vi "Cal Amplitude and Phase.vi"(1 "Inst Types":T1[](array[typedef]), 6 "Channel ID":string[](array[string]), 7 "Test Ch Indices":i32[](array[numeric]), 8 "Reference Ch Index":i32) -> (0 "Valid Indices":i32[](array[numeric]), 3 "Ch Values":dbl[](array[numeric]), 5 "Ch Names":string[](array[string]))   [LabVIEW 2022 SP3]
uses:
  Controls/Inst_type.ctl
  Globals/Meas_global.vi
  <vilib>/measure/matone.llb/Extract Single Tone Information 1 Chan.vi
  <vilib>/measure/NI_MAPro.lvlib
panel:
  out "Ref Freq FFT":dbl
  out "detected frequency Ref":dbl format="%.2p"
  out "detected frequency":dbl format="%.2p"
  out "Ref Freq Hz Tone":dbl
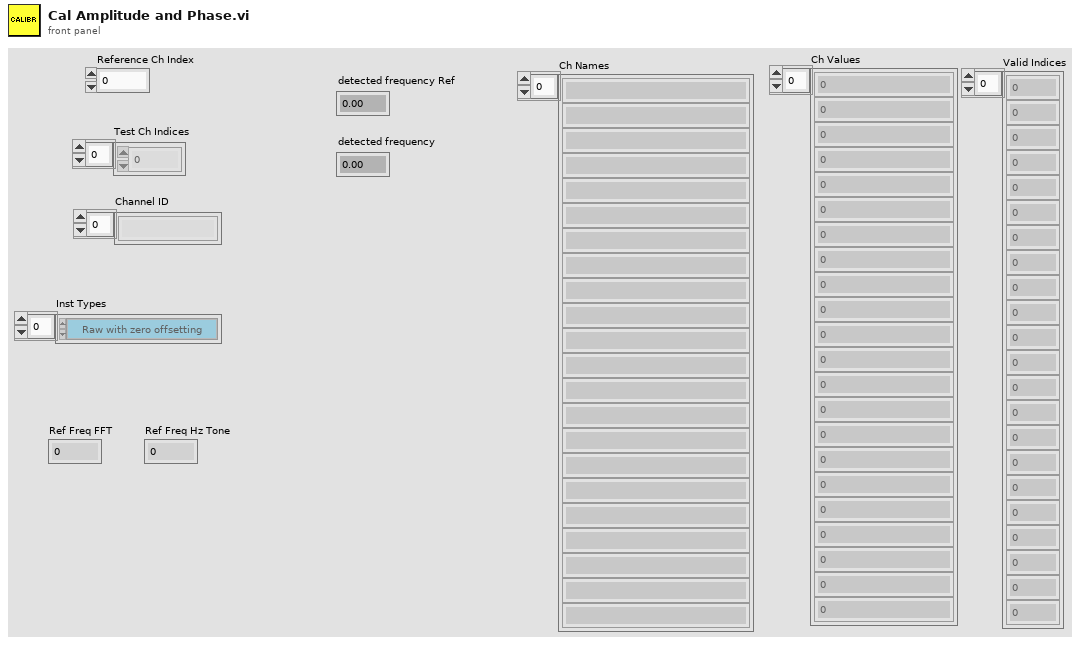
[diagram p1: front panel]
types:
  T1 = typedef "Inst_type.ctl" = enum16{"Raw voltage", "Raw with zero offsetting", "Propeller anemometer", "Pressure Transducer", "Pitot-static tube", "Hot wire", "Cross wire 1", "Cross wire 2", "Generic Linear", "Generic Polynomial", "Generic BackPoly", "Fast FID", "Thermocouple", "Cold wire", "Pulsed Wire", "LDA Vel", "LDA Tran time", "LDA Arr time", "Microphone"}
  T2 = typedef "Time_Trace_Cluster.ctl" = cluster{"Weighting":dbl[], "Voltage":dbl[], "Eng Values":dbl[]}
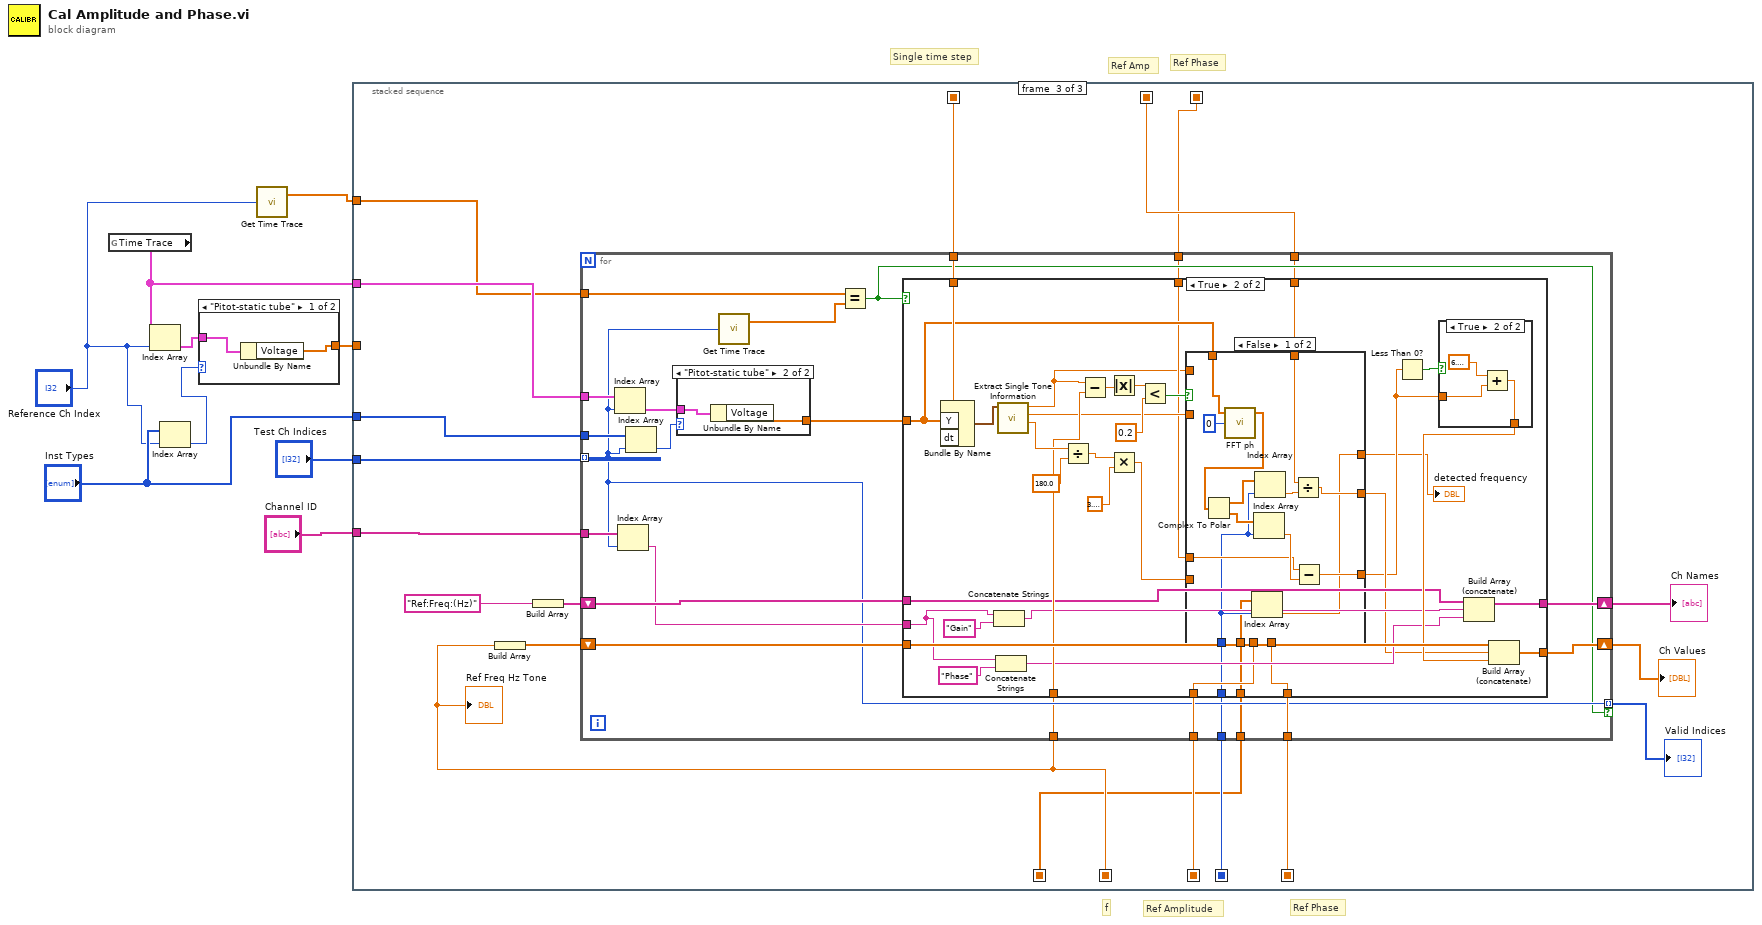
[diagram p0: block diagram]
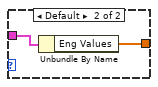
[diagram p2: hidden frame]
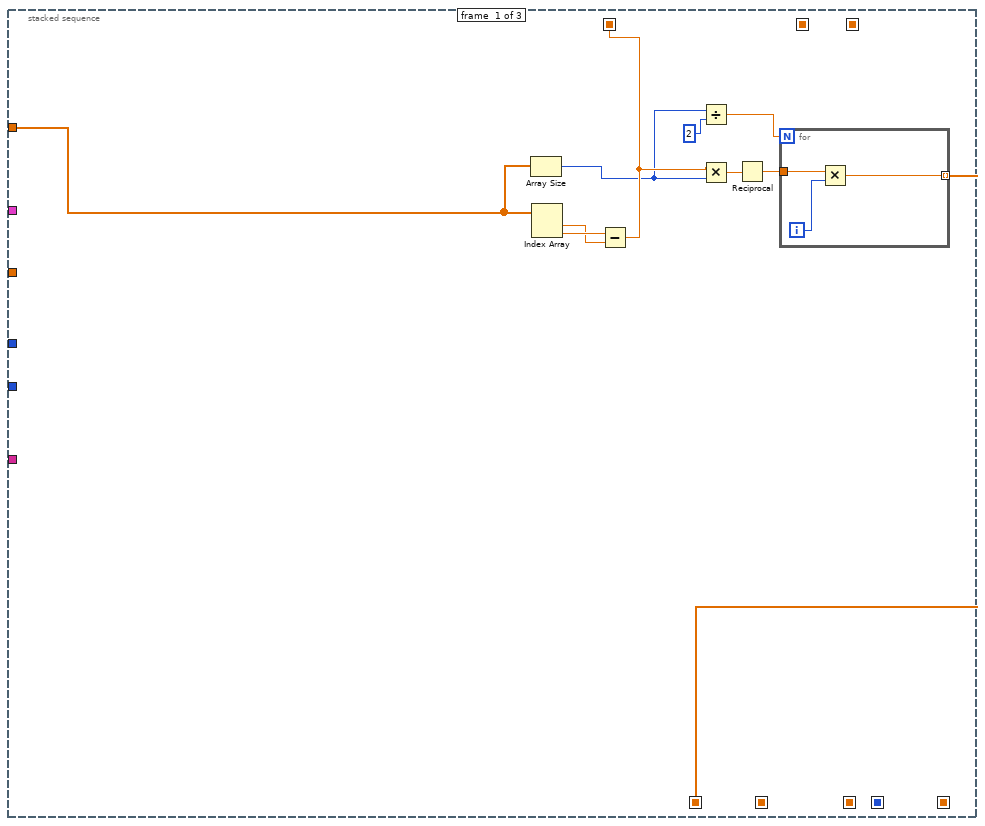
[diagram p3: hidden frame]
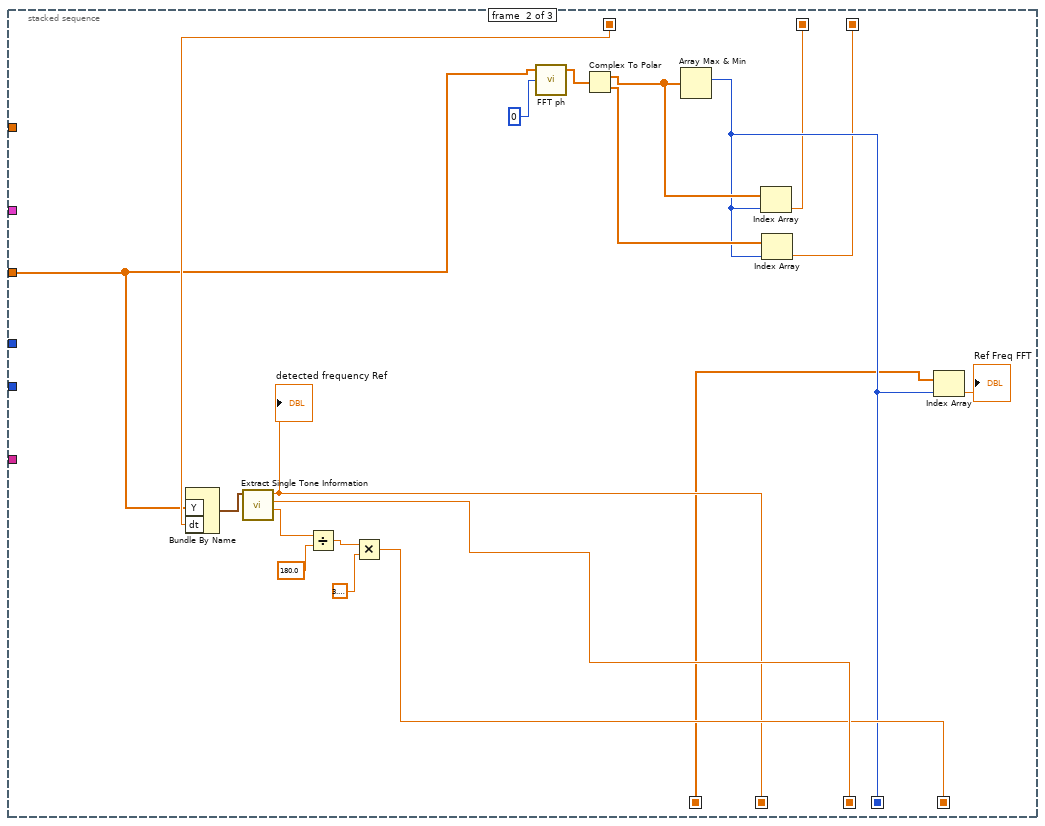
[diagram p4: hidden frame]
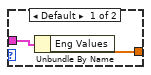
[diagram p5: hidden frame]
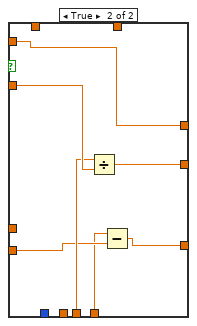
[diagram p7: hidden frame]
diagram:
  # "Ref Phase"
  # "Ref Amp"
  # "Single time step"
  # "Ref Phase"
  # "Ref Amplitude"
  # "f"
  n1 = global read "Meas_global.vi" "Time Trace"() -> (w7:T2[])
  n2 = Index Array(array=w7, index="Reference Ch Index") -> (element=w9:T2)
  n3 = Index Array(array="Inst Types", index="Reference Ch Index") -> (element=w4:T1)
  n4 = case shown="\"Pitot-static tube\"" w4 {
    tunnel: w9 -> [w11 w13]
    tunnel: [w10 w12] -> w8
    frame "Pitot-static tube" {
      n5 = Unbundle By Name(w11) -> ("Voltage"=w10:dbl[])
    }
    frame Default {
      n6 = Unbundle By Name(w13) -> ("Eng Values"=w12:dbl[])
    }
  }
  n7 = call "Get Time Trace.vi"("Channel Index"="Reference Ch Index") -> ("Time (s)"=w1:dbl[])  [unwired: 1 out]
  n8 = stacked-sequence {
    seq-local: [_ w38 _] -> [_ _ w50]
    seq-local: [_ w40 _] -> [_ _ w62]
    seq-local: [_ w39 _] -> [_ _ w61]
    seq-local: [w20 _ _] -> [_ w41 w51]
    seq-local: [w14 _ _] -> [_ w30 w46]
    seq-local: [_ w31 _] -> [_ _ w49]
    seq-local: [_ w27 _] -> [_ _ w47]
    seq-local: [_ w28 _] -> [_ _ w48]
    tunnel: w1 -> [w21 _ w63]
    tunnel: w8 -> [_ w33 _]
    tunnel: w7 -> [_ _ w64]
    tunnel: "Channel ID" -> [_ _ w54]
    tunnel: "Test Ch Indices" -> [_ _ w53]
    tunnel: "Inst Types" -> [_ _ w52]
    frame #0 {
      n9 = Array Size(array=w21) -> (size(s)=w18:i32)
      n10 = Index Array(array=w21) -> (element #1=w22:dbl, element #2=w23:dbl)  [unwired: 2 in]
      n11 = Subtract(x=w23, y=w22) -> (x-y=w20:dbl)
      n12 = Divide(x=w18, y=2) -> (x/y=w16:dbl)
      n13 = Multiply(x=w20, y=w18) -> (x*y=w19:dbl)
      n14 = Reciprocal(x=w19) -> (1/x=w15:dbl)
      n15 = for {
        N: w16 -> [_]
        tunnel: w15 -> [w26]
        tunnel: [w24] -> w14 mode=indexing
        i -> [w25]
        n16 = Multiply(x=w26, y=w25) -> (x*y=w24:dbl)
      }
    }
    frame #1 {
      n17 = Bundle By Name("Y"=w33, "dt"=w41) -> (w45:waveform(dbl))  [unwired: 1 in]
      n18 = call-poly <vilib>:"Extract Single Tone Information.vi"("time signal in"=w45) -> ("detected phase (deg)"=w37:dbl, "detected amplitude"=w40:dbl, "detected frequency"=w38:dbl)  [unwired: 5 in, 3 out]
      "detected frequency Ref" <- w38
      n19 = Divide(x=w37, y=180.0) -> (x/y=w43:dbl)
      n20 = Multiply(x=w43, y=3.141592653589793) -> (x*y=w39:dbl)
      n21 = call "FFT ph.vi"("Loop Index"=0, "Array"=w33) -> ("FFT {X}"=w32:cdb[])  [unwired: 2 in, 1 out]
      n22 = Complex To Polar(r * e^(i*theta)=w32) -> (r=w36:dbl[], theta=w35:dbl[])
      n23 = Array Max & Min(array=w36) -> (max index (indices)=w31:i32)  [unwired: 3 out]
      n24 = Index Array(array=w36, index=w31) -> (element=w28:dbl)
      n25 = Index Array(array=w35, index=w31) -> (element=w27:dbl)
      n26 = Index Array(array=w30, index=w31) -> (element=→"Ref Freq FFT":dbl)
    }
    frame #2 {
      n27 = Build Array(w50) -> (w58:dbl[])
      n28 = Build Array("Ref:Freq:(Hz)") -> (w56:string[])
      n29 = for {
        tunnel: w64 -> [w87]
        tunnel: w53 -> [w73] mode=indexing
        tunnel: w63 -> [w86]
        tunnel: w62 -> [w84]
        tunnel: w61 -> [w83]
        shift-right: [w81] -> w59
        shift-left: w58 -> [w82]
        tunnel: w54 -> [w80]
        shift-right: [w77] -> w60
        shift-left: w56 -> [w79]
        tunnel: [w73] -> w55 mode=indexing if=w69
        tunnel: w52 -> [w74]
        tunnel: w51 -> [w71]
        tunnel: w50 -> [w70]
        tunnel: w49 -> [w68]
        tunnel: w48 -> [w67]
        tunnel: w47 -> [w66]
        tunnel: w46 -> [w65]
        n30 = Index Array(array=w87, index=w73) -> (element=w76:T2)
        n31 = Index Array(array=w80, index=w73) -> (element=w78:string)
        n32 = Index Array(array=w74, index=w73) -> (element=w75:T1)
        n33 = case shown="\"Pitot-static tube\"" w75 {
          tunnel: [w89 w91] -> w85
          tunnel: w76 -> [w88 w90]
          frame Default {
            n34 = Unbundle By Name(w88) -> ("Eng Values"=w89:dbl[])
          }
          frame "Pitot-static tube" {
            n35 = Unbundle By Name(w90) -> ("Voltage"=w91:dbl[])
          }
        }
        n36 = call "Get Time Trace.vi"("Channel Index"=w73) -> ("Time (s)"=w72:dbl[])  [unwired: 1 out]
        n37 = Equal?(x=w86, y=w72) -> (x = y?=w69:bool)
        n38 = case shown="True" w69 {
          tunnel: w85 -> [_ w100]
          tunnel: w84 -> [_ w105]
          tunnel: w83 -> [_ w102]
          tunnel: w82 -> [w93 w128]
          tunnel: [w93 w127] -> w81
          tunnel: w79 -> [w92 w111]
          tunnel: w78 -> [_ w126]
          tunnel: [w92 w110] -> w77
          tunnel: w71 -> [_ w120]
          tunnel: w70 -> [_ w115]
          tunnel: w68 -> [_ w99]
          tunnel: w67 -> [_ w98]
          tunnel: w66 -> [_ w97]
          tunnel: w65 -> [_ w94]
          frame False {
          }
          frame True {
            n39 = Bundle By Name("Y"=w100, "dt"=w120) -> (w121:waveform(dbl))  [unwired: 1 in]
            n40 = Concatenate Strings(w126, "Gain" ("string")) -> (w109:string)
            n41 = Concatenate Strings(w126, "Phase" ("string")) -> (w108:string)
            n42 = call-poly <vilib>:"Extract Single Tone Information.vi"("time signal in"=w121) -> ("detected phase (deg)"=w119:dbl, "detected amplitude"=w106:dbl, "detected frequency"=w95:dbl)  [unwired: 5 in, 3 out]
            n43 = Divide(x=w119, y=180.0) -> (x/y=w117:dbl)
            n44 = Subtract(x=w95, y=w115) -> (x-y=w114:dbl)
            n45 = Absolute Value(x=w114) -> (abs(x)=w113:dbl)
            n46 = Multiply(x=w117, y=3.141592653589793) -> (x*y=w103:dbl)
            n47 = Less?(x=w113, y=0.2) -> (x < y?=w107:bool)
            n48 = case shown="False" w107 {
              tunnel: w106 -> [_ w149]
              tunnel: w105 -> [_ w148]
              tunnel: [w137 w147] -> w104
              tunnel: w103 -> [_ w146]
              tunnel: w102 -> [_ w145]
              tunnel: [w134 w144] -> w101
              tunnel: w100 -> [w140 _]
              tunnel: w99 -> [w131 _]
              tunnel: w98 -> [w135 _]
              tunnel: w97 -> [w132 _]
              tunnel: [w129 w143] -> w96
              tunnel: w95 -> [_ w143]
              tunnel: w94 -> [w130 _]
              frame False {
                n49 = call "FFT ph.vi"("Loop Index"=0, "Array"=w140) -> ("FFT {X}"=w141:cdb[])  [unwired: 2 in, 1 out]
                n50 = Complex To Polar(r * e^(i*theta)=w141) -> (r=w139:dbl[], theta=w138:dbl[])
                n51 = Index Array(array=w130, index=w131) -> (element=w129:dbl)
                n52 = Index Array(array=w138, index=w131) -> (element=w133:dbl)
                n53 = Index Array(array=w139, index=w131) -> (element=w136:dbl)
                n54 = Divide(x=w135, y=w136) -> (x/y=w137:dbl)
                n55 = Subtract(x=w132, y=w133) -> (x-y=w134:dbl)
              }
              frame True {
                n56 = Divide(x=w148, y=w149) -> (x/y=w147:dbl)
                n57 = Subtract(x=w145, y=w146) -> (x-y=w144:dbl)
              }
            }
            "detected frequency" <- w96
            n58 = Less Than 0?(x=w101) -> (x < 0?=w123:bool)
            n59 = case shown="True" w123 {
              tunnel: w101 -> [w150 w152]
              tunnel: [w150 w151] -> w122
              frame False {
              }
              frame True {
                n60 = Add(x=6.283185307179586, y=w152) -> (x+y=w151:dbl)
              }
            }
            n61 = Build Array (concatenate)(w111, w109, w108) -> (w110:string[])
            n62 = Build Array (concatenate)(w128, w104, w122) -> (w127:dbl[])
          }
        }
      }
      "Ch Names" <- w60
      "Ch Values" <- w59
      "Valid Indices" <- w55
      "Ref Freq Hz Tone" <- w50
    }
  }
